vi "GF_stop.vi"(7 "modIdTag":string="F1", 8 "error in (no error)":errorcluster, 11 "channel":refnum<k24>) -> (0 "error out":errorcluster)   [LabVIEW 2021]
uses:
  D:/psychometric_function_v2/lib/Grpc.Core.dll
  lib/Grpc.Core.dll
  D:/psychometric_function_v2/lib/FossilProtosSharp.dll
  lib/FossilProtosSharp.dll
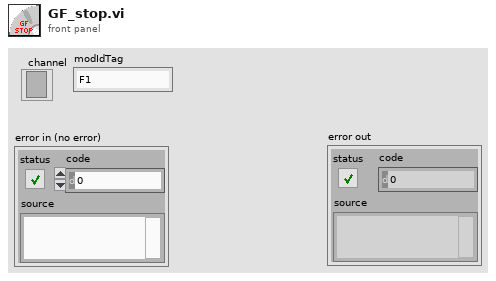
[diagram p1: front panel]
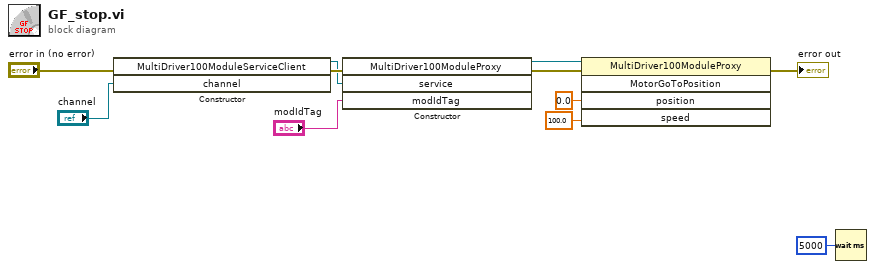
[diagram p0: block diagram]
diagram:
  n1 = constructor class="MultiDriver100ModuleServiceClie"(error in="error in (no error)", "channel"="channel") -> (reference out=w7:refnum<k24>, error out=w8:errorcluster)  [unwired: 2 in, 2 out]
  n2 = constructor class="MultiDriver100ModuleProxy"(error in=w8, "service"=w7, "modIdTag"="modIdTag") -> (reference out=w6:refnum<k24>, error out=w5:errorcluster)  [unwired: 2 in, 3 out]
  n3 = invoke class="MultiDriver100ModuleProxy" method="MotorGoToPosition"(reference=w6, error in=w5, "position"=sgl 0.0, "speed"=sgl 100.0) -> (error out=→"error out":errorcluster)  [unwired: 1 in, 4 out]
  n4 = Wait (ms)(milliseconds to wait=u32 5000) -> ()  [unwired: 1 out]
